vi "Support_BuildLogString.vi"(2 "log":T1[](array[typedef]) {"timestamp" format="%<%H:%M:%S%2u\n%Y/%m/%d>T"}, 5 "error in (no error)":errorcluster) -> (16 "LogString":string, 19 "error out":errorcluster)   [LabVIEW 2017]
doc: "Builds log string."
uses:
  Support_LogType.ctl
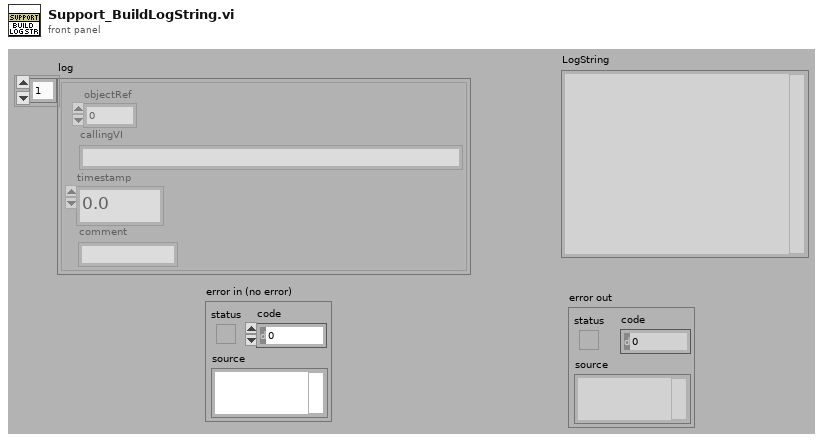
[diagram p1: front panel]
types:
  T1 = typedef "Support_LogType.ctl" = cluster{"objectRef":i32, "callingVI":string, "timestamp":dbl, "comment":string}
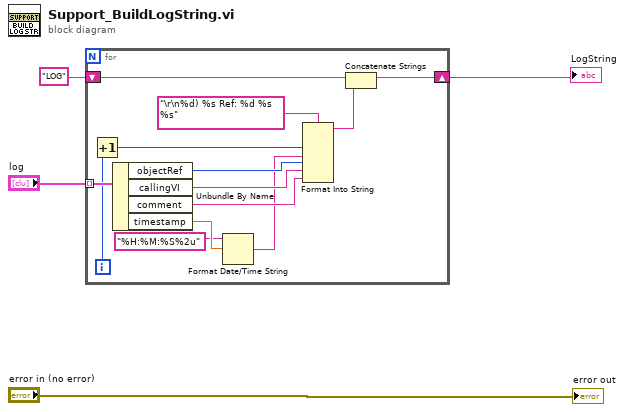
[diagram p0: block diagram]
diagram:
  n1 = for {
    tunnel: "log" -> [w17] mode=indexing
    shift-right: [w10] -> w1
    shift-left: "LOG" -> [w11]
    i -> [w14]
    n2 = Increment(x=w14) -> (x+1=w15:i32)
    n3 = Unbundle By Name(w17) -> ("objectRef"=w8:i32, "callingVI"=w9:string, "comment"=w16:string, "timestamp"=w7:dbl)
    n4 = Format Date/Time String(time format string (%c)="%H:%M:%S%2u", seconds (now)=w7) -> (date/time string=w5:string)  [unwired: 1 in]
    n5 = Format Into String(format string="\r\n%d) %s Ref: %d %s  %s", w15, w5, w8, w9, w16) -> (resulting string=w12:string)  [unwired: 2 in, 1 out]
    n6 = Concatenate Strings(w11, w12) -> (w10:string)
  }
  "LogString" <- w1
  "error out" <- "error in (no error)"
